vi "Stop Timer.vi"(0 "reference in":refnum<class "Timer.lvclass">, 5 "error in (no error)":errorcluster) -> (14 "reference out":refnum<class "Timer.lvclass">, 16 "Timer Time (min)":dbl, 17 "Timer Time (s)":dbl, 18 "Timer Time (ms)":u32, 19 "error out":errorcluster)   [LabVIEW 2017, in "Timer.lvclass"]
uses:
  Timer.lvclass
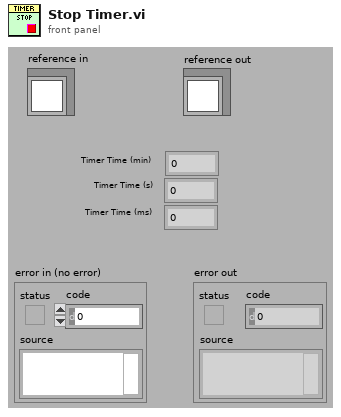
[diagram p1: front panel]
types:
  T1 = typedef "Timer.lvclass/ObjectAttributes.ctl" = cluster{"Timer is Timing":bool, "Timer Time (ms)":u32, "Timer VI Reference":refnum<vi>}
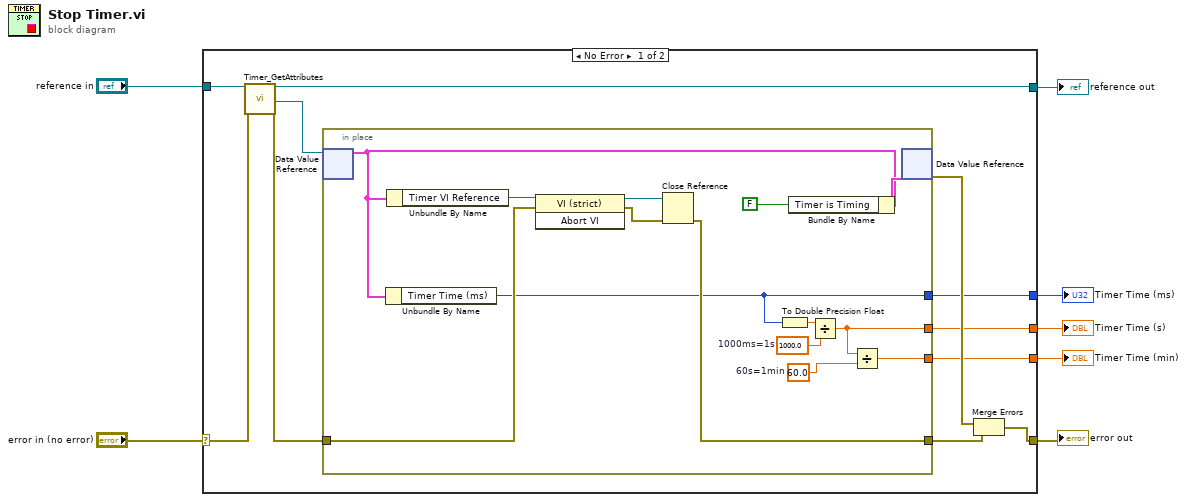
[diagram p0: block diagram]
diagram:
  n1 = case shown="No Error" "error in (no error)" {
    selector: "error in (no error)" -> [w17 w34]
    tunnel: [w15 w34] -> w6
    tunnel: [w11 w33] -> w4
    tunnel: "reference in" -> [w18 w33]
    tunnel: [w10 _] -> w3
    tunnel: [w9 _] -> w2
    tunnel: [w8 _] -> w1
    frame No Error {
      n2 = call "Timer_GetAttributes.vi"("reference in"=w18, "error in (no error)"=w17) -> ("reference out"=w11:refnum<class "Timer.lvclass">, "DataRef"=w14:refnum<data-value>, "error out"=w13:errorcluster)  [unwired: 14 in, 1 out]
      n3 = in-place {
        in-place-border: w13 -> [w28]
        in-place-border: [w26] -> w12
        in-place-border: [w23] -> w10
        in-place-border: [w22] -> w9
        in-place-border: [w21] -> w8
        w19 = 60.0  # 60s=1min
        w20 = 1000.0  # 1000ms=1s
        n4 = in-place-dvr #1(w14) -> (w25:T1)  [unwired: 1 out]
        n5 = Unbundle By Name(w25) -> ("Timer Time (ms)"=w23:u32)
        n6 = Unbundle By Name(w25) -> ("Timer VI Reference"=w30:refnum<vi>)
        n7 = invoke class="VI (strict)" method="Abort VI"(reference=w30, error in=w28) -> (reference out=w29:refnum<vi>, error out=w27:errorcluster)  [unwired: 1 in, 1 out]
        n8 = Close Reference(reference=w29, error in (no error)=w27) -> (error out=w26:errorcluster)
        n9 = To Double Precision Float(number=w23) -> (double precision float=w24:dbl)
        n10 = Bundle By Name(cluster=w25, "Timer is Timing"=FALSE) -> (w32:T1)
        n11 = Divide(x=w24, y=w20) -> (x/y=w22:dbl)
        n12 = Divide(x=w22, y=w19) -> (x/y=w21:dbl)
        n13 = in-place-dvr #1(w32) -> (w16:errorcluster)  [unwired: 1 out]
      }
      n14 = Merge Errors(w16, w12) -> (w15:errorcluster)
    }
    frame Error {
    }
  }
  "error out" <- w6
  "reference out" <- w4
  "Timer Time (ms)" <- w3
  "Timer Time (s)" <- w2
  "Timer Time (min)" <- w1
